vi "SortDefectLists.vi"(0 "No of bad strips":i32, 1 "Defect strips IN":i32[](array[numeric]), 2 "Defect flag array IN":i32[](array[numeric])) -> (3 "First defect No":i32[](array[numeric]), 4 "Last Defect No":i32[](array[numeric]), 5 "Defect Flag array OUT":i32[](array[numeric]), 6 "No of database entries":i32)   [LabVIEW 2013]
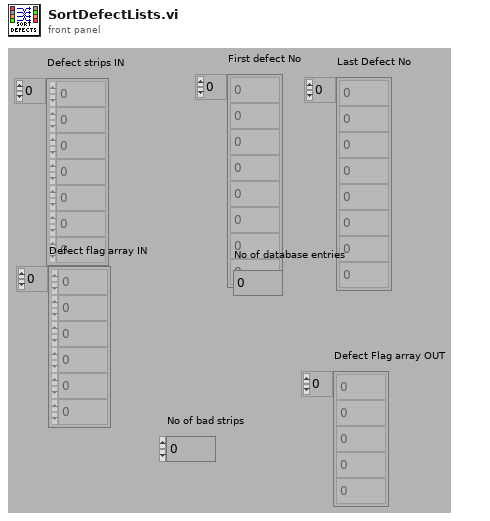
[diagram p1: front panel]
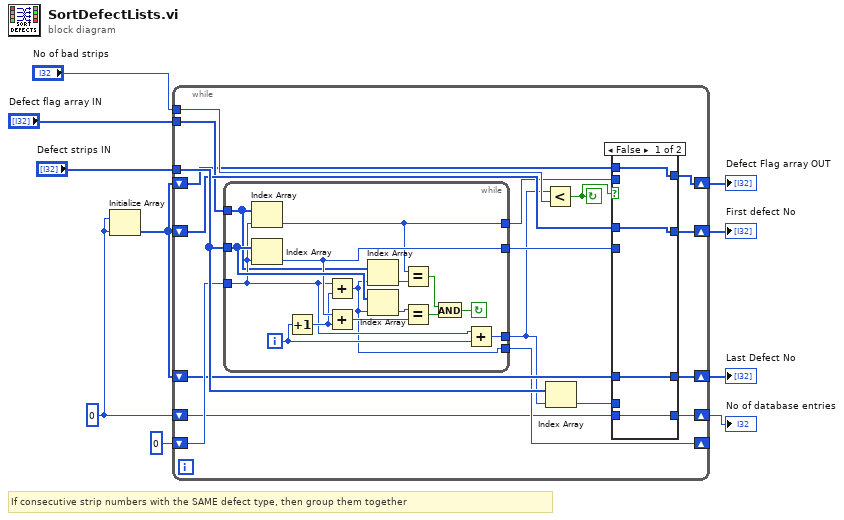
[diagram p0: block diagram]
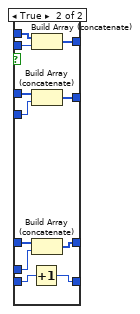
[diagram p2: hidden frame]
diagram:
  w6 = 0 ("Element Data")
  # "If consecutive strip numbers with the SAME defect type, then group them together"
  n1 = Initialize Array(w6, w6) -> (w3:i32[])
  n2 = while {
    tunnel: "Defect strips IN" -> [w28]
    shift-right: [w19] -> _
    shift-left: 0 -> [w27]
    shift-right: [w25] -> w9
    shift-left: w3 -> [w26]
    shift-right: [w21] -> w8
    shift-left: w3 -> [w23]
    tunnel: "No of bad strips" -> [w20]
    shift-right: [w15] -> w5
    shift-left: w6 -> [w16]
    tunnel: "Defect flag array IN" -> [w14]
    shift-right: [w12] -> w2
    shift-left: w3 -> [w13]
    stop <- w17 continue-if-true
    n3 = while {
      tunnel: w28 -> [w57]
      tunnel: w27 -> [w51]
      tunnel: [w56] -> w24
      tunnel: [w48] -> w19
      tunnel: [w52] -> w18
      tunnel: w14 -> [w49]
      tunnel: [w50] -> w11
      i -> [w53]
      stop <- w44 continue-if-true
      n4 = Index Array(array=w49, index=w51) -> (element=w50:i32)
      n5 = Index Array(array=w57, index=w51) -> (element=w56:i32)
      n6 = Increment(x=w53) -> (x+1=w55:i32)
      n7 = Add(x=w51, y=w55) -> (x+y=w48:i32)
      n8 = Add(x=w56, y=w55) -> (x+y=w58:i32)
      n9 = Index Array(array=w49, index=w48) -> (element=w47:i32)
      n10 = Index Array(array=w57, index=w48) -> (element=w54:i32)
      n11 = Equal?(x=w50, y=w47) -> (x = y?=w46:bool)
      n12 = Equal?(x=w54, y=w58) -> (x = y?=w45:bool)
      n13 = And(x=w46, y=w45) -> (x .and. y?=w44:bool)
      n14 = Add(x=w51, y=w53) -> (x+y=w52:i32)
    }
    n15 = Less?(x=w18, y=w20) -> (x < y?=w17:bool)
    n16 = Index Array(array=w28, index=w18) -> (element=w22:i32)
    n17 = case shown="False" w17 {
      tunnel: w26 -> [w32 w43]
      tunnel: [w32 w42] -> w25
      tunnel: w24 -> [_ w41]
      tunnel: w23 -> [w31 w40]
      tunnel: w22 -> [_ w39]
      tunnel: [w31 w38] -> w21
      tunnel: w16 -> [w30 w37]
      tunnel: [w30 w36] -> w15
      tunnel: w13 -> [w29 w35]
      tunnel: [w29 w34] -> w12
      tunnel: w11 -> [_ w33]
      frame False {
      }
      frame True {
        n18 = Increment(x=w37) -> (x+1=w36:i32)
        n19 = Build Array (concatenate)(w35, w33) -> (w34:i32[])
        n20 = Build Array (concatenate)(w43, w41) -> (w42:i32[])
        n21 = Build Array (concatenate)(w40, w39) -> (w38:i32[])
      }
    }
  }
  "First defect No" <- w9
  "Last Defect No" <- w8
  "No of database entries" <- w5
  "Defect Flag array OUT" <- w2
